vi "espInit.vi"(2 "error in (no error)":errorcluster, 3 "Axis":i32, 4 "RefNum":refnum<vi>, 5 "VISA resource name in":refnum<visa-resource-name>) -> (0 "error out":errorcluster, 1 "VISA resource name out":refnum<visa-resource-name>)   [LabVIEW 2014]
uses:
  ESP301/Newport ESP301.lvlib
panel:
  in  "ESP Cluster":T1 {"Set Velocity" min=0.0 max=0.2 format="%1.4f"}
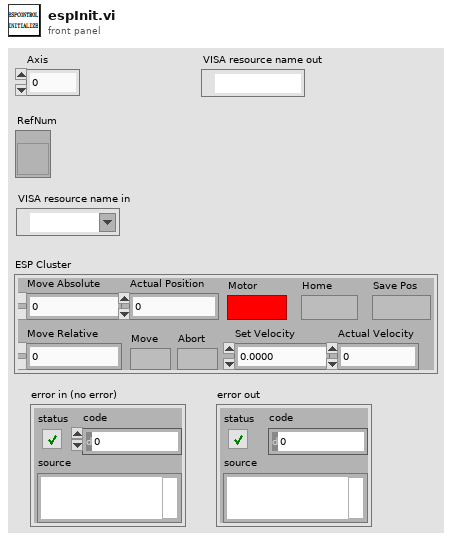
[diagram p1: front panel]
types:
  T1 = cluster{"Move Absolute":dbl, "Actual Position":dbl, "Motor":bool, "Home":bool, "Set Velocity":dbl, "Move Relative":dbl, "Actual Velocity":dbl, "Move":bool, "Save Pos":bool, "Abort":bool}
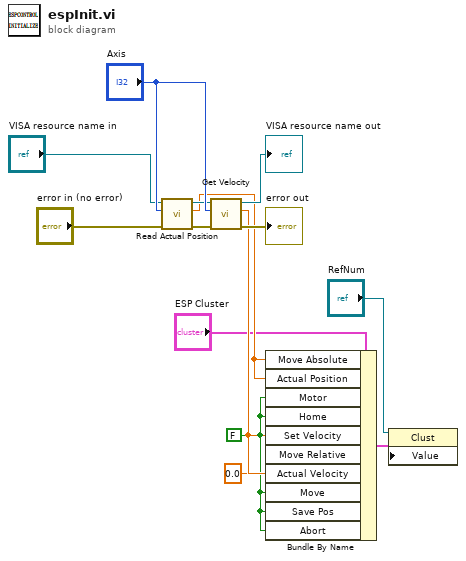
[diagram p0: block diagram]
diagram:
  w3 = FALSE
  n1 = call <instrlib>:"Read Actual Position.vi"("error in (no error)"="error in (no error)", "Axis (1)"="Axis", "VISA resource name"="VISA resource name in") -> ("error out"=w9:errorcluster, "Position (units)"=w7:dbl, "VISA resource name out"=w8:refnum<visa-resource-name>)  [unwired: 2 in]
  n2 = call "Get Velocity.vi"("error in (no error)"=w9, "Axis (1)"="Axis", "VISA resource name"=w8) -> ("error out"=→"error out":errorcluster, "Velocity (units/s)"=w11:dbl, "VISA resource name out"=→"VISA resource name out":refnum<visa-resource-name>)  [unwired: 2 in]
  n3 = Bundle By Name(cluster="ESP Cluster", "Move Absolute"=w7, "Actual Position"=w7, "Motor"=w3, "Home"=w3, "Set Velocity"=w11, "Move Relative"=0.0, "Actual Velocity"=w11, "Move"=w3, "Save Pos"=w3, "Abort"=w3) -> (w14:T1)
  n4 = property class="Clust"(reference="RefNum", "Value"=w14) -> ()  [unwired: 1 in, 2 out]
